vi "NotifyObserver_Single.vi"(8 "error in":errorcluster, 9 "ObservableDataValue":variant, 10 "ObservableDataName":string, 11 "IstanceName":string) -> (0 "error out":errorcluster)   [LabVIEW 2025, in "ObserverClass.lvlib"]
doc: "Send Notification to all the Observer"
uses:
  ObserverClass.lvlib
  ObserverClass/Controls/observerControl.ctl
  ObserverClass/ObserverClass.lvclass
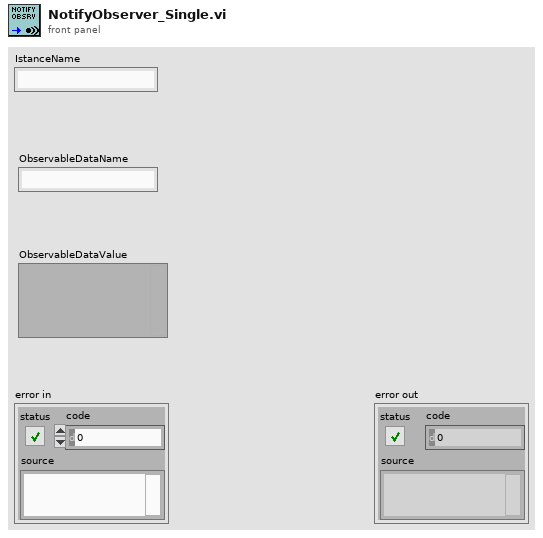
[diagram p1: front panel]
types:
  T1 = enum16{"Get", "Set", "Init", "Remove", "Destroy"}
  T2 = typedef "ObserverClass.lvlib/ObserverClass.lvclass/observerControl.ctl" = cluster{"ObservableName":string, "ObservableValue":variant, "SenderName":string}
  T3 = map{string, cluster{"ObserverEvent":refnum<user-event>, "ObserverNr":u64, "Value":variant}}
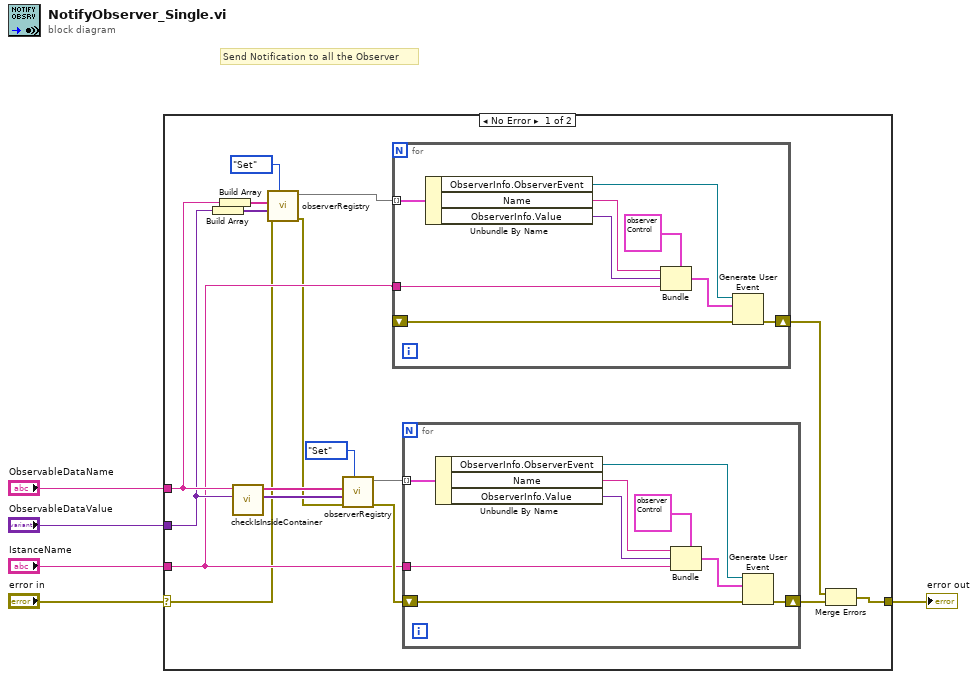
[diagram p0: block diagram]
diagram:
  # "Send Notification to all the Observer"
  n1 = case shown="No Error" "error in" {
    selector: "error in" -> [w8 w41]
    tunnel: "ObservableDataName" -> [w14 _]
    tunnel: "ObservableDataValue" -> [w13 _]
    tunnel: "IstanceName" -> [w10 _]
    tunnel: [w7 w41] -> w5
    frame No Error {
      n2 = Build Array(w13) -> (w11:variant[])
      n3 = Build Array(w14) -> (w12:string[])
      n4 = call "checkIsInsideContainer.vi"("ObservableValue"=w13, "ObservableName"=w14) -> ("ObservableValue out"=w17:variant[], "ObservableName out"=w18:string[])  [unwired: 7 in, 1 out]
      n5 = call "observerRegistry.vi"("Action"=T1."Set", "error in"=w8, "ObservableValue"=w11, "ObservableName"=w12) -> ("error out"=w9:errorcluster, "Observable out"=w15:T3)  [unwired: 5 in, 1 out]
      n6 = call "observerRegistry.vi"("Action"=T1."Set", "error in"=w9, "ObservableValue"=w17, "ObservableName"=w18) -> ("error out"=w19:errorcluster, "Observable out"=w21:T3)  [unwired: 5 in, 1 out]
      n7 = for {
        tunnel: w15 -> [w31] mode=indexing
        tunnel: w10 -> [w26]
        shift-right: [w23] -> w6
        shift-left: _ -> [w24]
        n8 = Unbundle By Name(w31) -> ("ObserverInfo.ObserverEvent"=w30:refnum<user-event>, "Name"=w27:string, "ObserverInfo.Value"=w25:variant)
        n9 = Bundle(cluster=T2 {"ObservableName"="", "ObservableValue"=variant, "SenderName"=""} ("event data"), "ObservableName"=w27, "ObservableValue"=w25, "SenderName"=w26) -> (w29:T2)
        n10 = Generate User Event(user event=w30, event data cluster=w29, error in=w24) -> (error out=w23:errorcluster)  [unwired: 1 in, 1 out]
      }
      n11 = for {
        tunnel: w21 -> [w40] mode=indexing
        tunnel: w10 -> [w35]
        shift-right: [w32] -> w20
        shift-left: w19 -> [w33]
        n12 = Unbundle By Name(w40) -> ("ObserverInfo.ObserverEvent"=w39:refnum<user-event>, "Name"=w36:string, "ObserverInfo.Value"=w34:variant)
        n13 = Bundle(cluster=T2 {"ObservableName"="", "ObservableValue"=variant, "SenderName"=""} ("event data"), "ObservableName"=w36, "ObservableValue"=w34, "SenderName"=w35) -> (w38:T2)
        n14 = Generate User Event(user event=w39, event data cluster=w38, error in=w33) -> (error out=w32:errorcluster)  [unwired: 1 in, 1 out]
      }
      n15 = Merge Errors(w6, w20) -> (w7:errorcluster)
    }
    frame Error {
    }
  }
  "error out" <- w5
